vi "Set Stop Trigger.vi"   [LabVIEW 2020, in "NI_VS Data Logging API.lvlib"]
doc: "Specifies a trigger condition on which to stop logging data. You also can specify whether to continue logging channel data for a set period of time after the trigger condition occurs.\n\nYou must manually select the polymorphic instance to use."
uses:
  <vilib>/NI VeriStand/Execution/DataLogging/NI_VS Data Logging API.lvlib
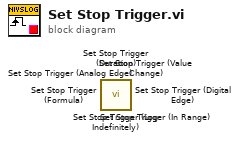
[diagram p0: block diagram]
diagram:
  n1 = call <vilib>:"Set Stop Trigger (Log Indefinitely).vi"() -> ()  [unwired: 10 in, 2 out]
  n2 = call <vilib>:"Set Stop Trigger (Value Change).vi"() -> ()  [unwired: 10 in, 2 out]
  n3 = call <vilib>:"Set Stop Trigger (Formula).vi"() -> ()  [unwired: 10 in, 2 out]
  n4 = call <vilib>:"Set Stop Trigger (Digital Edge).vi"() -> ()  [unwired: 10 in, 2 out]
  n5 = call <vilib>:"Set Stop Trigger (Analog Edge).vi"() -> ()  [unwired: 10 in, 2 out]
  n6 = call <vilib>:"Set Stop Trigger (Duration).vi"() -> ()  [unwired: 10 in, 2 out]
  n7 = call <vilib>:"Set Stop Trigger (In Range).vi"() -> ()  [unwired: 10 in, 2 out]
